vi "Get Class Private Data.vi"(8 "error in (no error)":errorcluster {"code" format="Error %.0f"}, 11 "Class Documentation In":refnum<class "Class Documentation.lvclass">) -> (0 "error out":errorcluster {"code" format="Error %.0f"}, 2 "Class Private Data":T1[](array[typedef]), 3 "Class Documentation Out":refnum<class "Class Documentation.lvclass">)   [LabVIEW 2023, in "VIDoc Parsing.lvlib" / "Class Documentation.lvclass"]
uses:
  Class Documentation.lvclass
  TypeDefs/Controls Info Cluster.ctl
  <vilib>/picture/picture.llb/imagedata.ctl
  <vilib>/Utility/miscctls.llb/LVKeyTypeDef.ctl
  Class Documentation.lvclass/Class Documentation.ctl
  VIDoc Parsing.lvlib
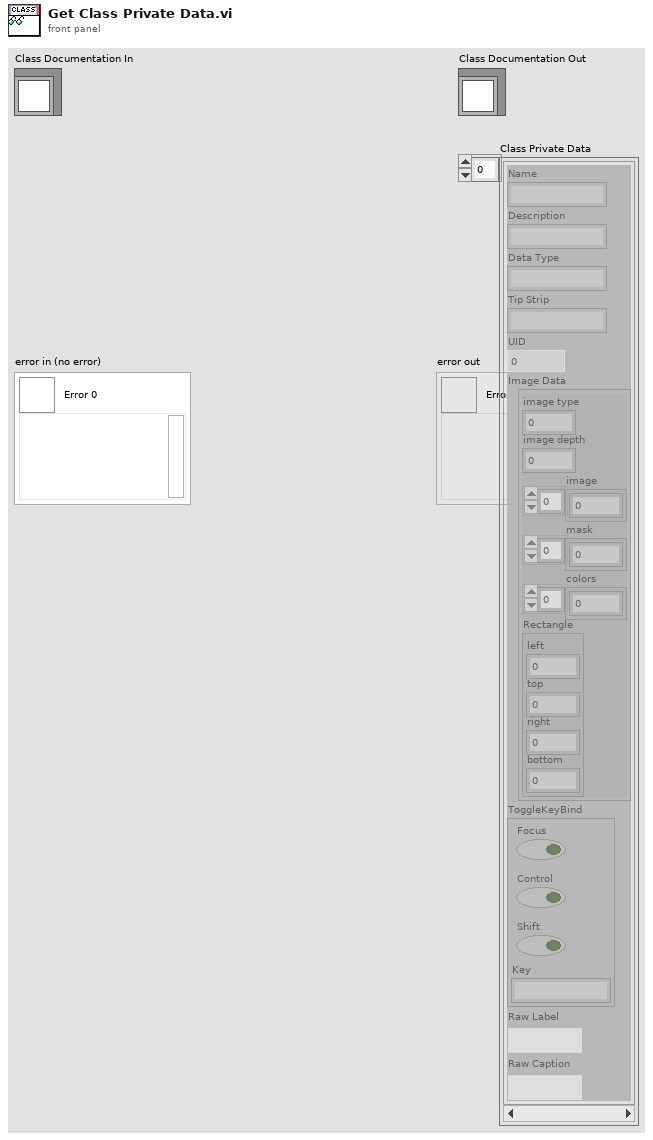
[diagram p1: front panel]
types:
  T1 = typedef "VIDoc Parsing.lvlib/Controls Info Cluster.ctl" = cluster{"Name":string, "Description":string, "Data Type":string, "Tip Strip":string, "UID":i32, "Image Data":T2, "ToggleKeyBind":T3, "Raw Label":string, "Raw Caption":string}
  T2 = typedef "imagedata.ctl" = cluster{"image type":i32, "image depth":i32, "image":u8[], "mask":u8[], "colors":u32[], "Rectangle":cluster{"left":i16, "top":i16, "right":i16, "bottom":i16}}
  T3 = typedef "LVKeyTypeDef.ctl" = cluster{"Focus":bool, "Control":bool, "Shift":bool, "Key":string}
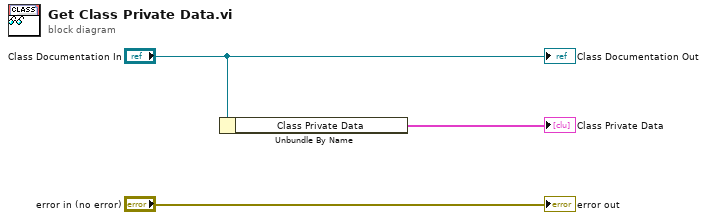
[diagram p0: block diagram]
diagram:
  n1 = Unbundle By Name("Class Documentation In") -> ("Class Private Data"=→"Class Private Data":T1[])
  "error out" <- "error in (no error)"
  "Class Documentation Out" <- "Class Documentation In"
